vi "DigitalTriggeredAudioNoiseVolumeCtrl.vi"() -> ()   [LabVIEW 2010]
uses:
  <vilib>/DAQmx/read.llb/DAQmx Read (Digital 1D Bool NChan 1Samp 1Line).vi
  <vilib>/DAQmx/read.llb/DAQmx Read (Counter 1D DBL 1Chan NSamp).vi
  <vilib>/DAQmx/create/channels.llb/DAQmx Create Channel (CI-Pulse Width).vi
  <vilib>/DAQmx/create/channels.llb/DAQmx Create Channel (DI-Digital Input).vi
  <vilib>/sound2/lvsound2.llb/Sound Output Write (DBL Single).vi
  <vilib>/daqmx/miscellaneous.llb/DAQmx Fill In Error Info.vi
  <vilib>/measure/NI_MAPro.lvlib
  <vilib>/Analysis/NI_AALBase.lvlib
panel:
  out "duty cycle":dbl
  out "start frequency":dbl
  out "triggered":bool
  in  "duration (sec)":dbl=2.0
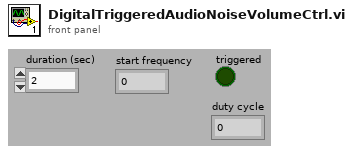
[diagram p1: front panel]
types:
  T1 = typedef "Sound Output Task ID.ctl" = u32
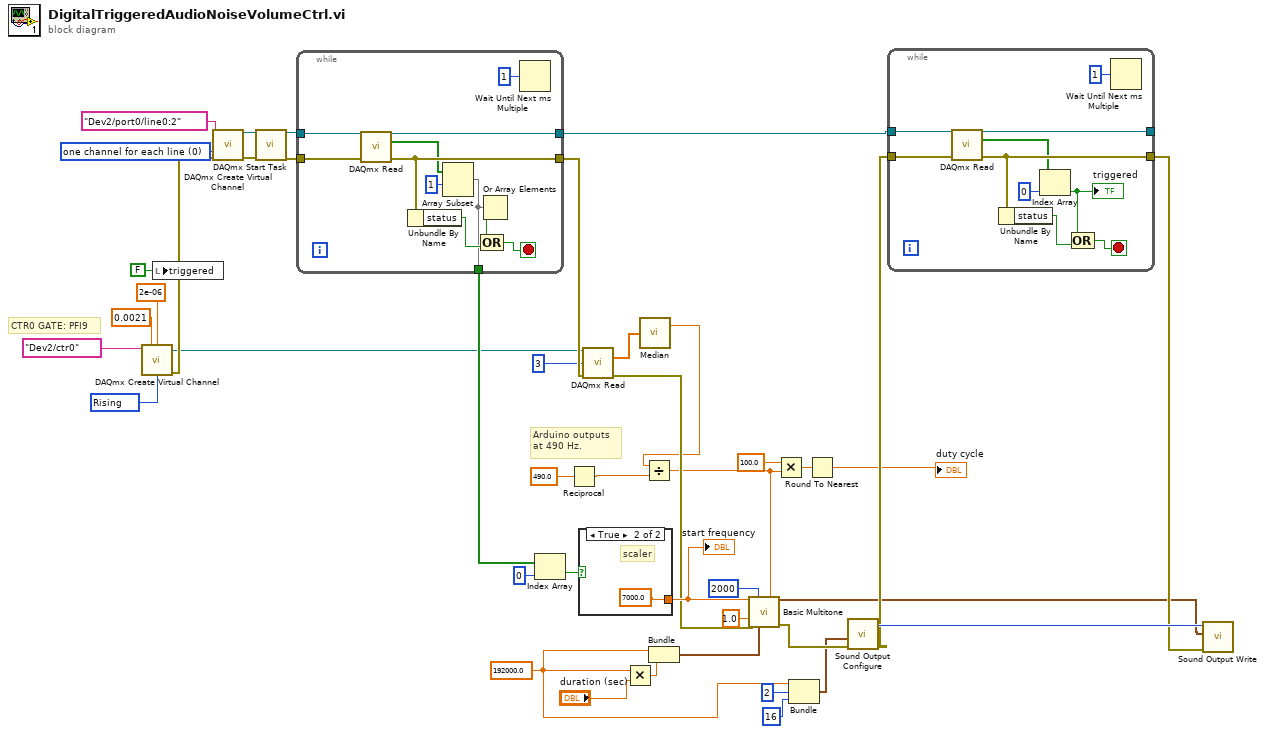
[diagram p0: block diagram]
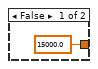
[diagram p2: hidden frame]
diagram:
  w4 = 10280 items=["Rising"=10280, "Falling"=10171] ("starting edge")
  w22 = 192000.0 ("x")
  w42 = 0 items=["one channel for each line", "one channel for all lines"] ("line grouping")
  # "Arduino outputs\nat 490 Hz."
  # "CTR0 GATE: PFI9"
  n1 = call-poly <vilib>:"DAQmx Create Virtual Channel.vi"("maximum value"=0.0021, "minimum value"=2e-06, "counter"=tag "Dev2/ctr0", "starting edge"=w4) -> ("task out"=w9:refnum<k21>, "error out"=w14:errorcluster)  [unwired: 10 in]
  n2 = local write "triggered"(FALSE ("triggered")) -> ()
  n3 = call-poly <vilib>:"DAQmx Create Virtual Channel.vi"("lines"=tag "Dev2/port0/line0:2", "line grouping"=w42, "error in"=w14) -> ("task out"=w38:refnum<k21>, "error out"=w37:errorcluster)  [unwired: 11 in]
  n4 = call <vilib>:"DAQmx Start Task.vi"("task/channels in"=w38, "error in"=w37) -> ("task out"=w36:refnum<k21>, "error out"=w35:errorcluster)  [unwired: 12 in]
  n5 = while {
    tunnel: w35 -> [w54]
    tunnel: [w51] -> w13
    tunnel: w36 -> [w50]
    tunnel: [w49] -> w34
    tunnel: [w44] -> w29
    stop <- w53 stop-if-true
    n6 = call-poly <vilib>:"DAQmx Read.vi"("task/channels in"=w50, "error in"=w54) -> ("task out"=w49:refnum<k21>, "data"=w45:bool[], "error out"=w51:errorcluster)  [unwired: 11 in]
    n7 = Unbundle By Name(w51) -> ("status"=w52:bool)
    n8 = Array Subset(array=w45, index=1) -> (w44:bool[])  [unwired: 1 in]
    n9 = Or Array Elements(Boolean array=w44) -> (logical OR=w47:bool)
    n10 = Compound Arithmetic op=OR(w47, w52) -> (w53:bool)
    n11 = Wait Until Next ms Multiple(millisecond multiple=u32 1 ("milliseconds to wait")) -> ()  [unwired: 1 out]
  }
  n12 = Index Array(array=w29, index=0) -> (element=w27:bool)
  n13 = Reciprocal(x=490.0) -> (1/x=w10:dbl)
  n14 = case shown="True" w27 {
    tunnel: [15000.0 ("start frequency") 7000.0 ("start frequency")] -> w26
    frame False {
    }
    frame True {
      # "scaler"
    }
  }
  "start frequency" <- w26
  n15 = call-poly <vilib>:"DAQmx Read.vi"("task/channels in"=w9, "number of samples per channel"=3, "error in"=w13) -> ("data"=w3:dbl[], "error out"=w12:errorcluster)  [unwired: 10 in, 1 out]
  n16 = Multiply(x=w22, y="duration (sec)") -> (x*y=w23:dbl)
  n17 = call <vilib>:"Median.vi"("X"=w3) -> ("median"=w2:dbl)  [unwired: 1 out]
  n18 = Divide(x=w2, y=w10) -> (x/y=w8:dbl)
  n19 = Bundle("x"=w22, w23) -> (w24:cluster{"x":dbl, dbl})  [unwired: 1 in]
  n20 = call <vilib>:"Basic Multitone.vi"("start frequency"=w26, "#tones"=2000, "amplitude"=w8, "delta frequency"=1.0, "error in (no error)"=w12, "sampling info"=w24) -> ("signal out"=w30:waveform(dbl), "error out"=w31:errorcluster)  [unwired: 6 in, 2 out]
  n21 = Multiply(x=100.0, y=w8) -> (x*y=w6:dbl)
  n22 = Bundle("x"=w22, 2, 16) -> (w19:cluster{"x":dbl, i32, i32})  [unwired: 1 in]
  n23 = Round To Nearest(number=w6) -> (nearest integer value=→"duty cycle":dbl)
  n24 = call <vilib>:"Sound Output Configure.vi"("error in (no error)"=w31, "sound format"=w19) -> ("error out"=w40:errorcluster, "task ID"=w43:T1)  [unwired: 8 in]
  n25 = while {
    tunnel: w40 -> [w66]
    tunnel: [w63] -> w39
    tunnel: w34 -> [w62]
    tunnel: [w61] -> _
    stop <- w65 stop-if-true
    n26 = call-poly <vilib>:"DAQmx Read.vi"("task/channels in"=w62, "error in"=w66) -> ("task out"=w61:refnum<k21>, "data"=w59:bool[], "error out"=w63:errorcluster)  [unwired: 11 in]
    n27 = Unbundle By Name(w63) -> ("status"=w64:bool)
    n28 = Index Array(array=w59, index=0) -> (element=w58:bool)
    "triggered" <- w58
    n29 = Compound Arithmetic op=OR(w58, w64) -> (w65:bool)
    n30 = Wait Until Next ms Multiple(millisecond multiple=u32 1 ("milliseconds to wait")) -> ()  [unwired: 1 out]
  }
  n31 = call-poly <vilib>:"Sound Output Write.vi"("error in (no error)"=w39, "data"=w30, "task ID"=w43) -> ()  [unwired: 7 in, 2 out]
